vi "2021_day5_task2.vi"() -> ()   [LabVIEW 2021]
panel:
  out "Total Overlap Points":i16
  out "result string":string
  out "Array 2":i32[][](array[numeric])
  out "Array":T1(array[cluster])
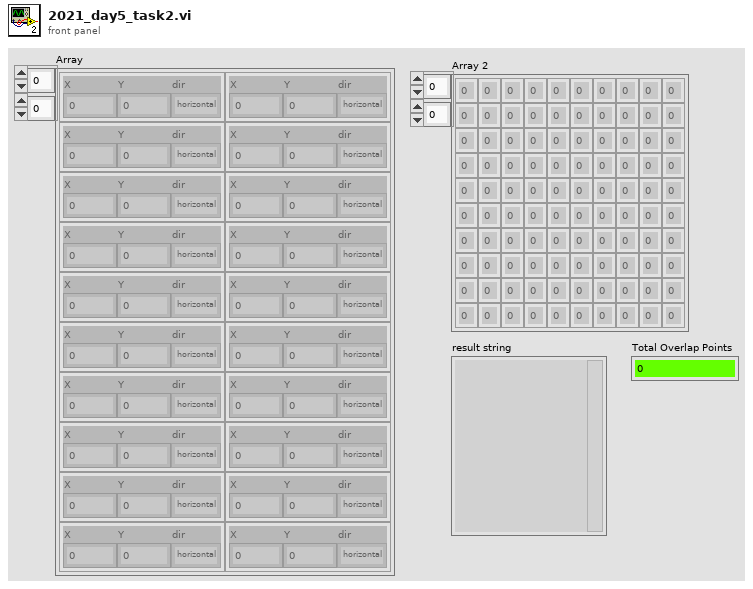
[diagram p1: front panel]
types:
  T1 = cluster{"X":i32, "Y":i32, "dir":enum16{"horizontal", "vertical"}}[][]
  T2 = cluster{"X":i32, "Y":i32, "dir":enum16{"horizontal", "vertical"}}
  T3 = cluster{"X":i32, "Y":i32, "dir":enum16{"horizontal", "vertical"}}[]
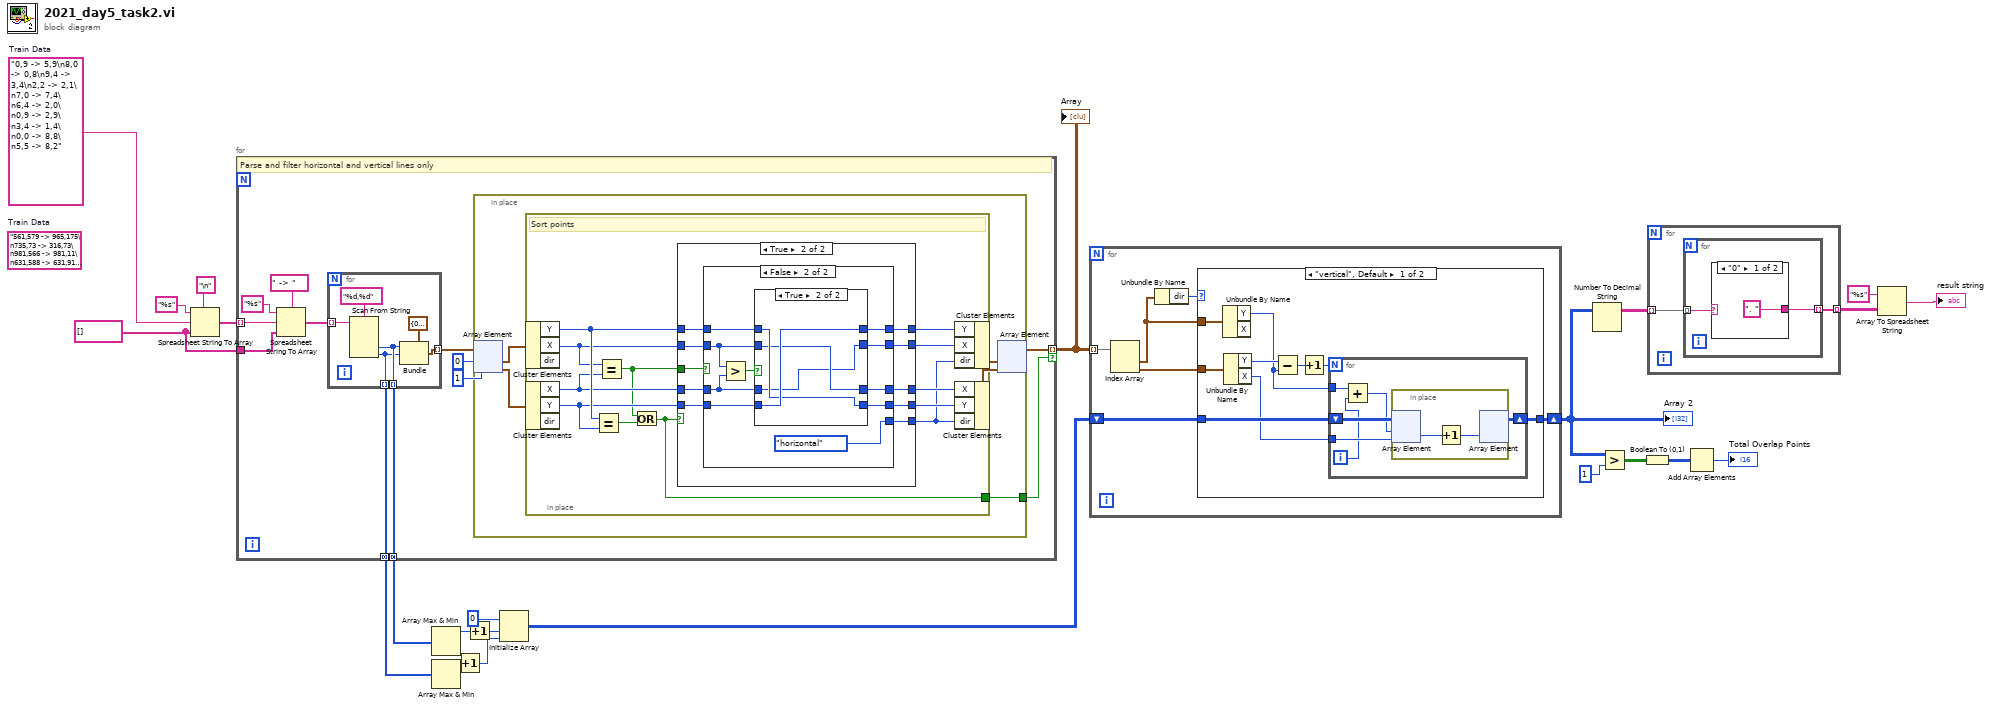
[diagram p0: block diagram]
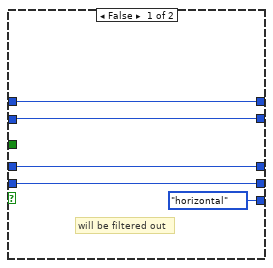
[diagram p3: hidden frame]
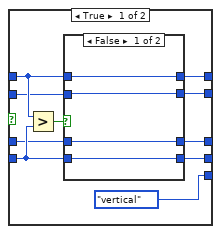
[diagram p4: hidden frame]
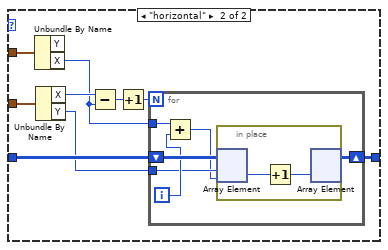
[diagram p7: hidden frame]
diagram:
  (unwired) "561,579 -> 965,175\n735,73 -> 316,73\n981,566 -> 981,11\n631,588 -> 631,910\n919,964 -> 70,115\n122,463 -> 261,602\n502,248 -> 774,248\n636,797 -> 797,958\n444,815 -> 444,554\n734,97 -> 734,210\n871,692 -> 368,692\n842,261 -> 606,261\n332,43 -> 206,43\n371,220 -> 18,573\n594,782 -> 127,782\n952,953 -> 72,73\n13,143 -> 755,885\n827,741 -> 827,168\n65,84 -> 839,858\n299,598 -> 299,588\n478,76 -> 607,76\n656,748 -> 61,153\n566,447 -> 857,447\n497,19 -> 310,206\n354,721 -> 538,721\n124,17 -> 124,339\n105,595 -> 843,595\n686,902 -> 919,669\n683,183 -> 776,183\n415,45 -> 415,942\n16,852 -> 843,25\n945,954 -> 23,32\n935,174 -> 485,624\n712,297 -> 792,297\n495,90 -> 497,90\n836,259 -> 836,988\n12,59 -> 916,963\n72,648 -> 72,185\n625,400 -> 507,282\n809,206 -> 809,538\n472,909 -> 472,213\n847,162 -> 189,162\n178,233 -> 178,777\n404,276 -> 404,516\n943,178 -> 400,721\n882,429 -> 882,920\n12,976 -> 900,88\n33,53 -> 958,53\n104,37 -> 609,542\n207,736 -> 800,143\n331,454 -> 331,715\n956,52 -> 26,982\n189,544 -> 189,368\n194,258 -> 451,258\n75,383 -> 75,642\n770,861 -> 915,716\n300,330 -> 300,683\n649,175 -> 344,175\n948,25 -> 42,931\n245,313 -> 748,816\n677,126 -> 677,204\n507,948 -> 507,88\n343,229 -> 343,677\n946,933 -> 472,459\n830,403 -> 830,660\n626,651 -> 626,213\n828,932 -> 828,487\n792,101 -> 216,101\n870,111 -> 50,931\n770,464 -> 290,944\n264,700 -> 941,23\n894,846 -> 630,846\n19,40 -> 957,978\n911,425 -> 393,425\n26,594 -> 26,475\n754,287 -> 754,302\n105,483 -> 807,483\n25,902 -> 684,243\n300,164 -> 532,396\n79,346 -> 79,423\n649,234 -> 649,331\n113,115 -> 962,964\n251,50 -> 531,330\n908,177 -> 908,817\n905,106 -> 905,570\n958,55 -> 41,972\n985,984 -> 62,61\n794,802 -> 328,802\n984,273 -> 370,887\n271,758 -> 237,792\n443,534 -> 835,926\n367,762 -> 367,521\n527,737 -> 717,737\n89,921 -> 89,299\n521,279 -> 108,279\n810,344 -> 760,394\n292,944 -> 292,941\n265,471 -> 265,949\n923,378 -> 415,886\n125,656 -> 434,656\n51,460 -> 51,542\n297,178 -> 297,587\n432,122 -> 241,122\n916,855 -> 451,390\n48,838 -> 636,838\n802,659 -> 784,641\n316,961 -> 417,961\n342,675 -> 568,675\n345,60 -> 352,60\n495,595 -> 284,806\n111,975 -> 815,271\n315,239 -> 315,333\n14,16 -> 930,932\n380,373 -> 380,346\n212,141 -> 212,691\n415,555 -> 651,319\n497,565 -> 96,164\n902,451 -> 735,451\n118,751 -> 521,751\n923,680 -> 613,370\n641,897 -> 233,489\n804,447 -> 259,447\n556,751 -> 968,751\n409,638 -> 409,65\n512,50 -> 432,130\n28,25 -> 988,985\n563,888 -> 563,502\n912,691 -> 950,691\n592,934 -> 592,433\n465,886 -> 408,886\n928,547 -> 671,290\n486,953 -> 496,943\n942,943 -> 42,43\n672,759 -> 266,759\n587,195 -> 763,371\n95,354 -> 687,946\n890,280 -> 734,124\n945,906 -> 945,168\n306,952 -> 306,257\n143,160 -> 810,827\n988,407 -> 167,407\n274,472 -> 817,472\n252,113 -> 430,291\n294,767 -> 176,767\n456,142 -> 423,142\n908,107 -> 176,839\n255,278 -> 447,86\n100,44 -> 969,913\n899,184 -> 899,986\n872,877 -> 47,52\n122,786 -> 228,786\n132,777 -> 312,777\n242,86 -> 36,86\n726,671 -> 690,635\n386,859 -> 790,455\n468,62 -> 636,62\n920,869 -> 920,790\n610,66 -> 633,43\n428,962 -> 428,717\n935,881 -> 278,224\n314,204 -> 458,204\n906,515 -> 712,515\n332,223 -> 744,223\n707,802 -> 842,802\n775,36 -> 946,207\n906,206 -> 142,970\n534,312 -> 534,622\n26,687 -> 26,417\n758,258 -> 688,188\n830,591 -> 830,286\n856,182 -> 924,182\n78,755 -> 78,880\n157,726 -> 157,904\n316,30 -> 752,30\n958,977 -> 10,29\n831,813 -> 284,813\n472,843 -> 989,326\n133,99 -> 133,537\n161,540 -> 846,540\n176,739 -> 78,739\n28,33 -> 969,974\n65,160 -> 879,974\n355,943 -> 355,685\n893,512 -> 225,512\n789,565 -> 789,81\n253,832 -> 943,832\n372,716 -> 372,605\n781,293 -> 702,293\n469,497 -> 469,149\n692,499 -> 933,258\n477,548 -> 477,849\n131,894 -> 131,483\n934,765 -> 13,765\n830,55 -> 436,449\n615,496 -> 531,412\n78,634 -> 78,115\n205,586 -> 205,661\n871,742 -> 871,590\n218,223 -> 218,741\n56,897 -> 872,81\n30,886 -> 728,188\n369,877 -> 369,963\n202,55 -> 930,783\n251,131 -> 251,749\n498,313 -> 498,126\n688,876 -> 188,876\n147,968 -> 607,508\n400,693 -> 235,693\n206,853 -> 206,211\n401,158 -> 187,158\n35,957 -> 973,19\n517,822 -> 517,282\n836,492 -> 433,895\n751,114 -> 100,114\n80,359 -> 710,359\n302,871 -> 812,871\n853,159 -> 853,548\n351,663 -> 451,763\n895,260 -> 307,848\n369,455 -> 812,455\n936,594 -> 393,51\n55,696 -> 972,696\n422,804 -> 192,804\n110,893 -> 120,883\n747,645 -> 747,181\n636,344 -> 636,88\n15,949 -> 543,421\n985,948 -> 51,14\n164,435 -> 164,27\n30,966 -> 965,31\n600,472 -> 985,472\n119,161 -> 91,161\n180,521 -> 180,802\n98,70 -> 449,70\n157,190 -> 613,190\n816,501 -> 338,23\n387,219 -> 387,75\n115,579 -> 115,734\n26,153 -> 26,450\n733,783 -> 462,783\n19,893 -> 759,893\n646,726 -> 286,726\n631,139 -> 631,664\n490,668 -> 490,231\n282,958 -> 282,816\n338,55 -> 898,55\n891,420 -> 443,420\n222,917 -> 222,759\n302,430 -> 465,430\n946,49 -> 946,753\n101,971 -> 879,193\n329,122 -> 888,122\n524,714 -> 154,344\n89,769 -> 552,306\n749,680 -> 749,536\n161,510 -> 161,317\n143,608 -> 543,608\n677,526 -> 658,526\n348,956 -> 512,956\n851,973 -> 358,480\n850,247 -> 56,247\n284,274 -> 381,274\n855,944 -> 101,190\n338,102 -> 467,102\n225,875 -> 225,303\n120,944 -> 945,119\n485,386 -> 305,386\n321,866 -> 627,866\n44,207 -> 44,244\n514,763 -> 514,578\n617,930 -> 617,371\n963,838 -> 451,326\n813,904 -> 174,265\n901,983 -> 512,594\n979,929 -> 527,477\n533,383 -> 59,857\n871,724 -> 828,767\n174,133 -> 174,75\n686,911 -> 15,911\n361,406 -> 440,327\n759,284 -> 275,284\n231,431 -> 203,431\n759,673 -> 839,673\n914,897 -> 914,937\n598,643 -> 598,722\n697,297 -> 697,55\n735,918 -> 735,81\n375,538 -> 375,403\n868,86 -> 170,784\n390,142 -> 390,553\n569,564 -> 569,800\n514,276 -> 717,73\n756,768 -> 182,768\n349,428 -> 349,364\n370,386 -> 370,621\n191,224 -> 191,447\n672,983 -> 209,983\n281,854 -> 872,854\n898,959 -> 898,207\n961,597 -> 561,197\n965,837 -> 338,210\n120,675 -> 914,675\n401,661 -> 401,167\n706,536 -> 706,598\n856,337 -> 283,910\n980,535 -> 156,535\n941,888 -> 179,126\n585,47 -> 933,395\n481,435 -> 481,818\n989,978 -> 45,34\n693,332 -> 693,528\n863,605 -> 507,961\n586,429 -> 252,429\n37,61 -> 962,986\n952,26 -> 16,962\n926,492 -> 863,492\n661,110 -> 279,110\n524,879 -> 176,879\n298,424 -> 858,984\n498,627 -> 498,963\n468,608 -> 256,820\n61,491 -> 472,491\n38,922 -> 938,22\n361,938 -> 361,46\n567,981 -> 567,973\n399,575 -> 902,72\n618,740 -> 818,540\n79,115 -> 929,965\n612,972 -> 612,698\n217,626 -> 474,369\n961,593 -> 961,70\n287,450 -> 287,676\n703,45 -> 871,45\n756,778 -> 410,778\n960,970 -> 42,52\n254,513 -> 554,813\n620,339 -> 601,320\n650,344 -> 650,33\n597,349 -> 597,491\n761,106 -> 891,236\n323,846 -> 883,846\n678,190 -> 134,190\n400,848 -> 400,271\n198,68 -> 463,68\n522,805 -> 522,445\n979,134 -> 719,134\n584,493 -> 584,471\n635,10 -> 635,768\n867,795 -> 31,795\n157,824 -> 939,42\n354,381 -> 653,381\n45,628 -> 45,860\n959,870 -> 808,719\n587,810 -> 291,810\n248,34 -> 83,199\n656,505 -> 656,388\n966,90 -> 966,934\n957,834 -> 267,144\n690,367 -> 447,367\n153,948 -> 153,510\n467,260 -> 467,332\n69,43 -> 931,905\n913,92 -> 913,827\n226,504 -> 226,615\n21,737 -> 21,819\n391,289 -> 391,341\n566,639 -> 723,639\n160,824 -> 167,824\n77,69 -> 379,371\n756,864 -> 756,960\n315,569 -> 927,569\n964,864 -> 964,167\n136,277 -> 136,184\n524,450 -> 898,450\n971,903 -> 222,903\n962,958 -> 70,66\n525,570 -> 45,90\n164,352 -> 164,433\n703,61 -> 668,61\n289,136 -> 768,136\n50,65 -> 861,876\n676,199 -> 676,411\n294,370 -> 56,132\n299,840 -> 620,840\n845,776 -> 845,66\n61,18 -> 909,866\n738,670 -> 738,438\n974,618 -> 974,169\n669,800 -> 607,800\n935,427 -> 537,427\n441,898 -> 441,462\n490,768 -> 490,239\n275,788 -> 947,116\n650,412 -> 493,255\n382,89 -> 950,89\n865,194 -> 865,266\n977,677 -> 459,677\n128,18 -> 985,875\n199,646 -> 199,611\n666,149 -> 666,504\n129,539 -> 129,266\n332,364 -> 332,211\n619,132 -> 619,580\n426,69 -> 426,236\n123,334 -> 22,334\n792,57 -> 449,57\n33,976 -> 987,22\n221,614 -> 809,614\n245,379 -> 280,379\n895,238 -> 895,500\n957,423 -> 119,423\n917,50 -> 346,621\n183,263 -> 708,263\n452,174 -> 452,216\n404,681 -> 287,798\n931,54 -> 474,54\n815,264 -> 151,928\n736,507 -> 295,66\n200,160 -> 901,861\n709,975 -> 100,366\n126,468 -> 393,201\n822,627 -> 287,92\n101,285 -> 176,285\n250,581 -> 250,799\n257,446 -> 257,927\n436,423 -> 640,219\n468,229 -> 987,748\n394,245 -> 501,245\n37,931 -> 684,931\n123,54 -> 123,453\n75,364 -> 758,364\n256,62 -> 143,62\n933,299 -> 933,410\n313,887 -> 313,34\n453,833 -> 457,833\n614,87 -> 614,816\n48,113 -> 48,646\n977,571 -> 977,967\n982,989 -> 32,39\n773,749 -> 239,215\n983,989 -> 218,224\n885,606 -> 169,606\n63,53 -> 63,29\n96,870 -> 820,870\n544,895 -> 389,740\n61,246 -> 296,246\n812,82 -> 53,841\n749,399 -> 749,935\n882,168 -> 274,168\n566,673 -> 499,606\n572,558 -> 806,792\n923,79 -> 923,844\n875,416 -> 875,112\n393,18 -> 393,149\n389,844 -> 147,844\n207,157 -> 207,949\n467,644 -> 728,644\n36,29 -> 587,29\n448,370 -> 448,247\n43,283 -> 43,122\n709,837 -> 709,265\n294,273 -> 98,273\n625,869 -> 26,270\n156,26 -> 145,26\n393,544 -> 393,456\n708,536 -> 64,536\n324,519 -> 324,950\n138,788 -> 533,788\n117,818 -> 254,681\n953,766 -> 306,119\n669,325 -> 669,940\n421,416 -> 715,416\n886,101 -> 886,371\n786,656 -> 786,169\n123,641 -> 622,142\n658,504 -> 985,177\n440,505 -> 74,139\n300,616 -> 300,473\n265,729 -> 983,11\n501,396 -> 274,396\n877,123 -> 113,887\n544,78 -> 544,604\n287,944 -> 287,391\n766,854 -> 97,185\n959,49 -> 127,881\n715,727 -> 715,647\n339,557 -> 339,610\n19,133 -> 87,133\n872,94 -> 932,94\n966,935 -> 95,64\n137,942 -> 918,161\n162,718 -> 598,282\n256,18 -> 256,47\n597,658 -> 314,941\n817,685 -> 137,685\n20,14 -> 988,982\n970,916 -> 100,46\n672,152 -> 672,842\n468,825 -> 468,911\n673,731 -> 267,325"  # Train Data
  w20 = string[] [] ("array type (2D Dbl)")
  w1 = "0,9 -> 5,9\n8,0 -> 0,8\n9,4 -> 3,4\n2,2 -> 2,1\n7,0 -> 7,4\n6,4 -> 2,0\n0,9 -> 2,9\n3,4 -> 1,4\n0,0 -> 8,8\n5,5 -> 8,2"  # Train Data
  n1 = Spreadsheet String To Array(delimiter (Tab)="\n", format string="%s", spreadsheet string=w1, array type (2D Dbl)=w20) -> (array=w21:string[])
  n2 = for {
    tunnel: w21 -> [w34] mode=indexing
    tunnel: w20 -> [w32]
    tunnel: [w29] -> w19 mode=indexing if=w28
    tunnel: [w25] -> w17 mode=concatenating
    tunnel: [w24] -> w18 mode=concatenating
    # "Parse and filter horizontal and vertical lines only"
    n3 = Spreadsheet String To Array(delimiter (Tab)=" -> ", format string="%s", spreadsheet string=w34, array type (2D Dbl)=w32) -> (array=w31:string[])
    n4 = for {
      tunnel: w31 -> [w41] mode=indexing
      tunnel: [w39] -> w30 mode=indexing
      tunnel: [w37] -> w25 mode=indexing
      tunnel: [w36] -> w24 mode=indexing
      n5 = Scan From String(format string="%d,%d", input string=w41) -> (output 1=w37:i32, output 2=w36:i32)  [unwired: 4 in, 3 out]
      n6 = Bundle(cluster=T2 {"X"=0, "Y"=0, "dir"=enum."horizontal"}, "X"=w37, "Y"=w36) -> (w39:T2)  [unwired: 1 in]
    }
    n7 = in-place {
      in-place-border: [w44] -> w28
      n8 = in-place-array #1(w30, 0, 1) -> (w46:T2, w45:T2)
      n9 = in-place {
        in-place-border: [w48] -> w44
        # "Sort points"
        n10 = in-place-cluster #2(w46) -> ("Y"=w57:i32, "X"=w55:i32)  [unwired: 1 out]
        n11 = in-place-cluster #3(w45) -> ("X"=w54:i32, "Y"=w56:i32)  [unwired: 1 out]
        n12 = Equal?(x=w57, y=w56) -> (x = y?=w58:bool)
        n13 = Equal?(x=w55, y=w54) -> (x = y?=w49:bool)
        n14 = Or(x=w49, y=w58) -> (x .or. y?=w48:bool)
        n15 = case shown="True" w48 {
          tunnel: w57 -> [w63 w73]
          tunnel: w56 -> [w60 w72]
          tunnel: w55 -> [w62 w71]
          tunnel: w54 -> [w61 w70]
          tunnel: [w63 w69] -> w53
          tunnel: [w62 w68] -> w52
          tunnel: [w61 w67] -> w51
          tunnel: [w60 w66] -> w50
          tunnel: w49 -> [_ w65]
          tunnel: [enum16{"horizontal", "vertical"}."horizontal" ("dir") w64] -> w47
          frame False {
            # "will be filtered out"
          }
          frame True {
            n16 = case shown="False" w65 {
              tunnel: w73 -> [w83 w101]
              tunnel: w72 -> [w82 w100]
              tunnel: w71 -> [w80 w94]
              tunnel: w70 -> [w79 w93]
              tunnel: [w78 w98] -> w69
              tunnel: [w77 w97] -> w68
              tunnel: [w76 w96] -> w67
              tunnel: [w75 w95] -> w66
              tunnel: [enum16{"horizontal", "vertical"}."vertical" ("dir") enum16{"horizontal", "vertical"}."horizontal" ("dir")] -> w64
              frame True {
                n17 = Greater?(x=w83, y=w82) -> (0:w81:bool)
                n18 = case shown="False" w81 {
                  tunnel: w83 -> [w87 w90]
                  tunnel: w82 -> [w84 w91]
                  tunnel: w80 -> [w86 w89]
                  tunnel: w79 -> [w85 w88]
                  tunnel: [w87 w91] -> w78
                  tunnel: [w86 w88] -> w77
                  tunnel: [w85 w89] -> w76
                  tunnel: [w84 w90] -> w75
                  frame False {
                  }
                  frame True {
                  }
                }
              }
              frame False {
                n19 = Greater?(x=w94, y=w93) -> (0:w99:bool)
                n20 = case shown="True" w99 {
                  tunnel: w101 -> [w105 w108]
                  tunnel: w100 -> [w102 w109]
                  tunnel: w94 -> [w104 w107]
                  tunnel: w93 -> [w103 w106]
                  tunnel: [w105 w109] -> w98
                  tunnel: [w104 w106] -> w97
                  tunnel: [w103 w107] -> w96
                  tunnel: [w102 w108] -> w95
                  frame False {
                  }
                  frame True {
                  }
                }
              }
            }
          }
        }
        n21 = in-place-cluster #2("Y"=w53, "X"=w52, "dir"=w47) -> (w43:T2)
        n22 = in-place-cluster #3("X"=w51, "Y"=w50, "dir"=w47) -> (w42:T2)
      }
      n23 = in-place-array #1(w43, w42) -> (w29:T3)  [unwired: 2 out]
    }
  }
  "Array" <- w19
  n24 = Array Max & Min(array=w17) -> (max value=w15:i32)  [unwired: 3 out]
  n25 = Array Max & Min(array=w18) -> (max value=w14:i32)  [unwired: 3 out]
  n26 = Increment(x=w14) -> (x+1=w11:i32)
  n27 = Increment(x=w15) -> (x+1=w12:i32)
  n28 = Initialize Array(0, w12, w11) -> (w13:i32[][])
  n29 = for {
    tunnel: w19 -> [w115] mode=indexing
    shift-right: [w110] -> w6
    shift-left: w13 -> [w111]
    n30 = Index Array(array=w115) -> (element #1=w113:T2, element #2=w114:T2)  [unwired: 2 in]
    n31 = Unbundle By Name(w113) -> ("dir"=w112:enum16{"horizontal", "vertical"})
    n32 = case shown="\"vertical\", Default" w112 {
      tunnel: w114 -> [w124 w141]
      tunnel: w113 -> [w123 w140]
      tunnel: w111 -> [w122 w139]
      tunnel: [w121 w138] -> w110
      frame "vertical", Default {
        n33 = Unbundle By Name(w123) -> ("Y"=w117:i32)  [unwired: 1 out]
        n34 = Unbundle By Name(w124) -> ("Y"=w119:i32, "X"=w120:i32)
        n35 = Subtract(x=w119, y=w117) -> (x-y=w118:i32)
        n36 = Increment(x=w118) -> (x+1=w116:i32)
        n37 = for {
          N: w116 -> [_]
          shift-right: [w129] -> w121
          shift-left: w122 -> [w130]
          tunnel: w120 -> [w128]
          tunnel: w117 -> [w127]
          i -> [w126]
          n38 = Add(x=w127, y=w126) -> (x+y=w125:i32)
          n39 = in-place {
            n40 = in-place-array #4(w130, w125, w128) -> (w132:i32)
            n41 = Increment(x=w132) -> (x+1=w131:i32)
            n42 = in-place-array #4(w131) -> (w129:i32[][])  [unwired: 2 out]
          }
        }
      }
      frame "horizontal" {
        n43 = Unbundle By Name(w140) -> ("X"=w133:i32)  [unwired: 1 out]
        n44 = Unbundle By Name(w141) -> ("X"=w136:i32, "Y"=w137:i32)
        n45 = Subtract(x=w136, y=w133) -> (x-y=w135:i32)
        n46 = Increment(x=w135) -> (x+1=w134:i32)
        n47 = for {
          N: w134 -> [_]
          shift-right: [w146] -> w138
          shift-left: w139 -> [w147]
          tunnel: w137 -> [w143]
          tunnel: w133 -> [w145]
          i -> [w144]
          n48 = Add(x=w145, y=w144) -> (x+y=w142:i32)
          n49 = in-place {
            n50 = in-place-array #5(w147, w143, w142) -> (w149:i32)
            n51 = Increment(x=w149) -> (x+1=w148:i32)
            n52 = in-place-array #5(w148) -> (w146:i32[][])  [unwired: 2 out]
          }
        }
      }
    }
  }
  "Array 2" <- w6
  n53 = Number To Decimal String(number=w6) -> (decimal integer string=w5:string[][])  [unwired: 1 in]
  n54 = Greater?(x=w6, y=1) -> (0:w9:bool[][])
  n55 = Boolean To (0,1)(Boolean=w9) -> (0, 1=w8:i16[][])
  n56 = for {
    tunnel: w5 -> [w151] mode=indexing
    tunnel: [w150] -> w4 mode=indexing
    n57 = for {
      tunnel: w151 -> [w153] mode=indexing
      tunnel: [w152] -> w150 mode=indexing
      n58 = case shown="\"0\"" w153 {
        selector: w153 -> [_ w155]
        tunnel: [". " ("replace string (\"\")") w155] -> w152
        frame "0" {
        }
        frame "1", Default {
        }
      }
    }
  }
  n59 = Add Array Elements(numeric array=w8) -> (sum=→"Total Overlap Points":i16)
  n60 = Array To Spreadsheet String(array=w4, 3:"%s" ("format string")) -> (spreadsheet string=→"result string":string)  [unwired: 1 in]
